vi "_SSHTest.vi"() -> ()   [LabVIEW 2022 SP3]
panel:
  out "Reply":string
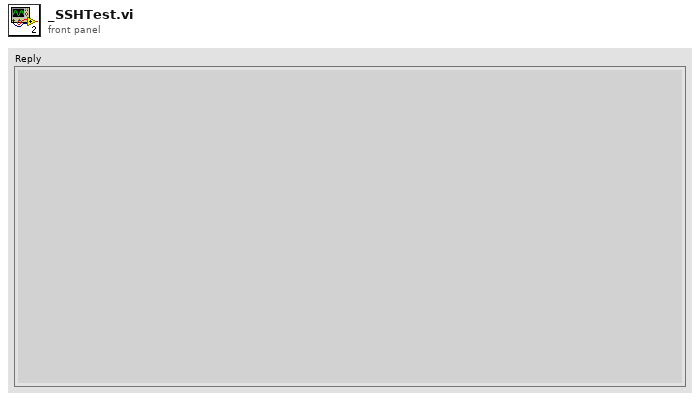
[diagram p1: front panel]
types:
  T1 = cluster{"IP Address":string, "Username":string, "password":string}
  T2 = typedef "PythonCtrl.ctl" = cluster{"session":refnum<k35>, "PyPath":path, "Processor":T3, "Port":string, "version":string}
  T3 = typedef "Processors.ctl" = enum16{"SPIKE", "Pi", "Pi_ssh", "OpenMV", "Dunio"}
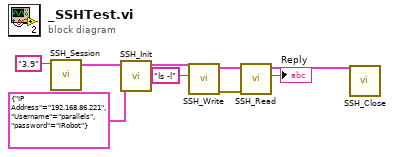
[diagram p0: block diagram]
diagram:
  n1 = call "SSH_Session.vi"("Python version"="3.9") -> ("Python"=w8:T2)  [unwired: 9 in, 1 out]
  n2 = call "SSH_Init.vi"("Raspberry Pi"=T1 {"IP Address"="192.168.86.221", "Username"="parallels", "password"="iRobot"}, "Python in"=w8) -> ("Python out"=w7:T2)  [unwired: 7 in, 2 out]
  n3 = call "SSH_Write.vi"("Text to write"="ls -l", "Python"=w7) -> ("error out"=w5:errorcluster, "Python"=w4:T2)  [unwired: 8 in]
  n4 = call "SSH_Read.vi"("error in (no error)"=w5, "Python"=w4) -> ("Reply"=→"Reply":string, "Python"=w2:T2)  [unwired: 7 in, 1 out]
  n5 = call "SSH_Close.vi"("Python"=w2) -> ()  [unwired: 9 in, 2 out]
